vi "LVClass_CorrectionDataManager SetInteractionMatrixPreferences.vi"(0 "CorrectionDataManager in":refnum<class "CorrectionDataManager.lvclass">, 5 "push_pull_value":T1, 11 "error in (no error)":errorcluster) -> (4 "CorrectionDataManager out":refnum<class "CorrectionDataManager.lvclass">, 15 "error out":errorcluster)   [LabVIEW 2020, in "CorrectionDataManager.lvclass"]
doc: "Calibrations preferences setter.\n\n--------------------------------------------------------------------------------\n\n<B>corrdata_managerIn </B> : CorrDataManager object.\n<B>corrdata_managerOut </B> : CorrDataManager object.\n<B>exp_type </B> : Type of calibration :\n * 0 : sequence of push-pull moves (each actuator is moved back then forth around its 0 position)\n * 1 : from file (user-defined experiments).\n<B>push_pull_value </B> : In case experiment type is \"push-pull\" (type 0), indicates the actuators\n displacement amplitude.\n<B>calibration_file_path </B> : In case experiment type is \"from file\" (type 1), path to the file containing\n the calibration steps.\n<B>ErrorIn </B> : Error\n<B>ErrorOut </B> : Error\n\n--------------------------------------------------------------------------------"
uses:
  CorrectionDataManager.lvclass
  InteractionMatrixAcquisitionParameters.ctl
  LVClass_CorrectionDataManager Read CorrectionDataManager.vi
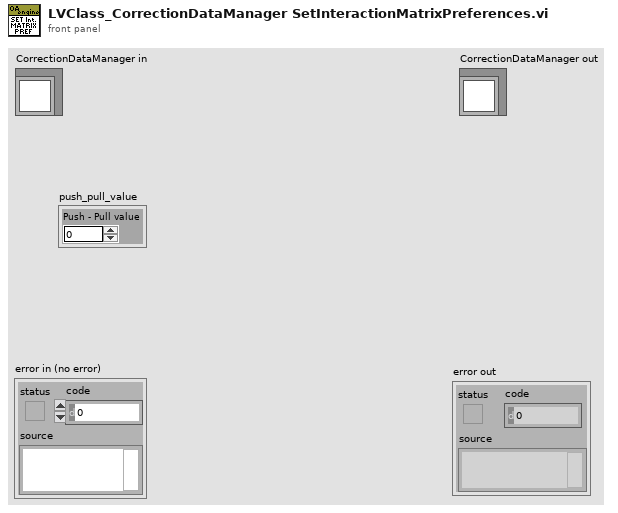
[diagram p1: front panel]
types:
  T1 = typedef "InteractionMatrixAcquisitionParameters.ctl" = cluster{"Push - Pull value":sgl}
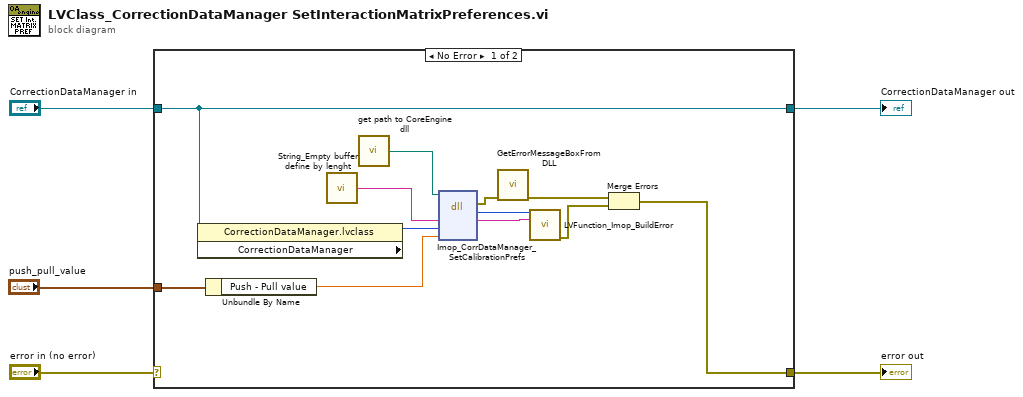
[diagram p0: block diagram]
diagram:
  n1 = case shown="No Error" "error in (no error)" {
    selector: "error in (no error)" -> [_ w19]
    tunnel: [w9 w19] -> w2
    tunnel: [w10 w18] -> w5
    tunnel: "CorrectionDataManager in" -> [w10 w18]
    tunnel: "push_pull_value" -> [w7 _]
    frame No Error {
      n2 = property class="CorrectionDataManager.lvclass"(reference=w10) -> ("CorrectionDataManager"=w8:i32)  [unwired: 1 in, 2 out]
      n3 = Unbundle By Name(w7) -> ("Push - Pull value"=w6:sgl)
      n4 = call "String_Empty buffer define by lenght.vi"() -> ("Empty buffer"=w15:string)  [unwired: 1 in]
      n5 = call "get path to CoreEngine dll.vi"() -> ("path to c_interface_vc100.dll"=w14:path)  [unwired: 12 in, 3 out]
      n6 = dll-call lib="D:/soft/HASO_v3/SVN_trunk/ImOpCoreEngine4_LV2011/DLLs/c_interface_vc100.dll" fn="Imop_CorrDataManager_SetCalibrationPrefs"(path in=w14, "message"=w15, "WavefrontCorrection"=w8, "push_pull_value"=w6) -> (error out=w13:errorcluster, "return type"=w17:i32, "message"=w16:string)  [unwired: 4 in, 1 out]
      n7 = call "GetErrorMessageBoxFromDLL.vi"("error IN"=w13) -> ("error OUT"=w12:errorcluster)  [unwired: 10 in]
      n8 = call "LVFunction_Imop_BuildError.vi"("code"=w17, "String to Prepend to source (\"\")"=w16) -> ("error out"=w11:errorcluster)  [unwired: 13 in]
      n9 = Merge Errors(w12, w11) -> (w9:errorcluster)
    }
    frame Error {
    }
  }
  "error out" <- w2
  "CorrectionDataManager out" <- w5
